vi "Read Front panel controls.vi"(8 "error in (no error)":errorcluster, 11 "PS Control Actor in":refnum<class "PS Control Actor.lvclass">) -> (0 "error out":errorcluster, 2 "Front panel controls":refnum<vi>[](array[refnum]), 3 "PS Control Actor out":refnum<class "PS Control Actor.lvclass">)   [LabVIEW 2019, in "PS Control Actor.lvlib" / "PS Control Actor.lvclass"]
uses:
  PS Control Actor.lvclass
  PS Control Actor.lvclass/PS Control Actor.ctl
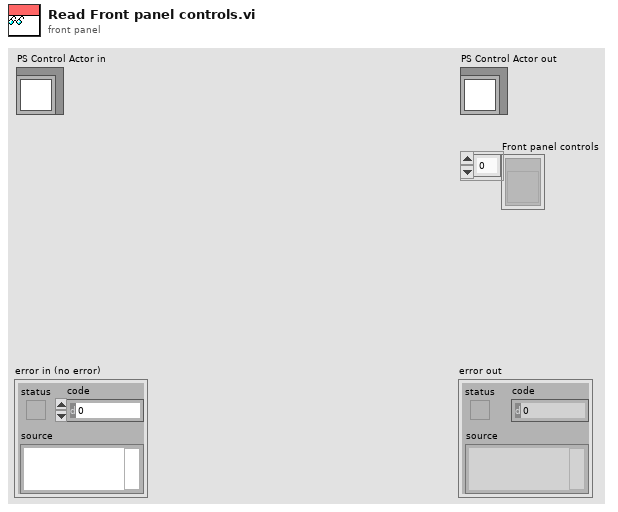
[diagram p1: front panel]
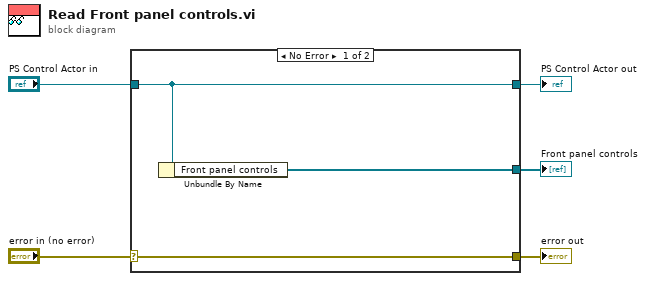
[diagram p0: block diagram]
diagram:
  n1 = case shown="No Error" "error in (no error)" {
    selector: "error in (no error)" -> [w8 w9]
    tunnel: [w8 w9] -> w4
    tunnel: [w7 w10] -> w2
    tunnel: "PS Control Actor in" -> [w7 w10]
    tunnel: [w6 _] -> w1
    frame No Error {
      n2 = Unbundle By Name(w7) -> ("Front panel controls"=w6:refnum<vi>[])
    }
    frame Error {
    }
  }
  "error out" <- w4
  "PS Control Actor out" <- w2
  "Front panel controls" <- w1
